vi "Hi_Port_TEST_SET.vi"(4 "itemiput":string, 5 "input":string, 6 "SEQ":i32, 7 "tpdata in":string[](array[string])) -> (3 "tpdata out":string[](array[string]))   [LabVIEW 2018]
panel:
  in  "Bar":bool
  out "布尔":bool
  in  "退出":bool
  out "out":string
  in  "Tab Control":enum32{"DataSetign", "RelaySeting"}(tab)
  in  "Address":string(combo)="PCI-1713"
  in  "Start board number":string(combo)="1"
  in  "Test Type":string(combo)="0"
  in  "Output Current Max.Spec":string="*" caption="MAX"
  in  "Output Current Min.Spec":string="*" caption="MIN"
  in  "延时时间(ms)2":string="0" caption="Delay Time (ms)"
  in  "备注":string
  in  "H 2":bool[](array[boolean])
  in  "L 2":bool[](array[boolean])
  in  "H":bool[](array[boolean])
  in  "L":bool[](array[boolean])
  in  "L 3":bool[](array[boolean])
  in  "H 3":bool[](array[boolean])
  in  "L 4":bool[](array[boolean])
  in  "H 4":bool[](array[boolean])
  in  "Cancel":bool
  in  "OK":bool
  # "EditTestData"
  # "9-16位输出"
  # "17-24位输出"
  # "25-32位输出"
  # "33-40位输出"
  # "41-48位输出"
  # "49-56位输出"
  # "57-64位输出"
  # "1-8位输出"
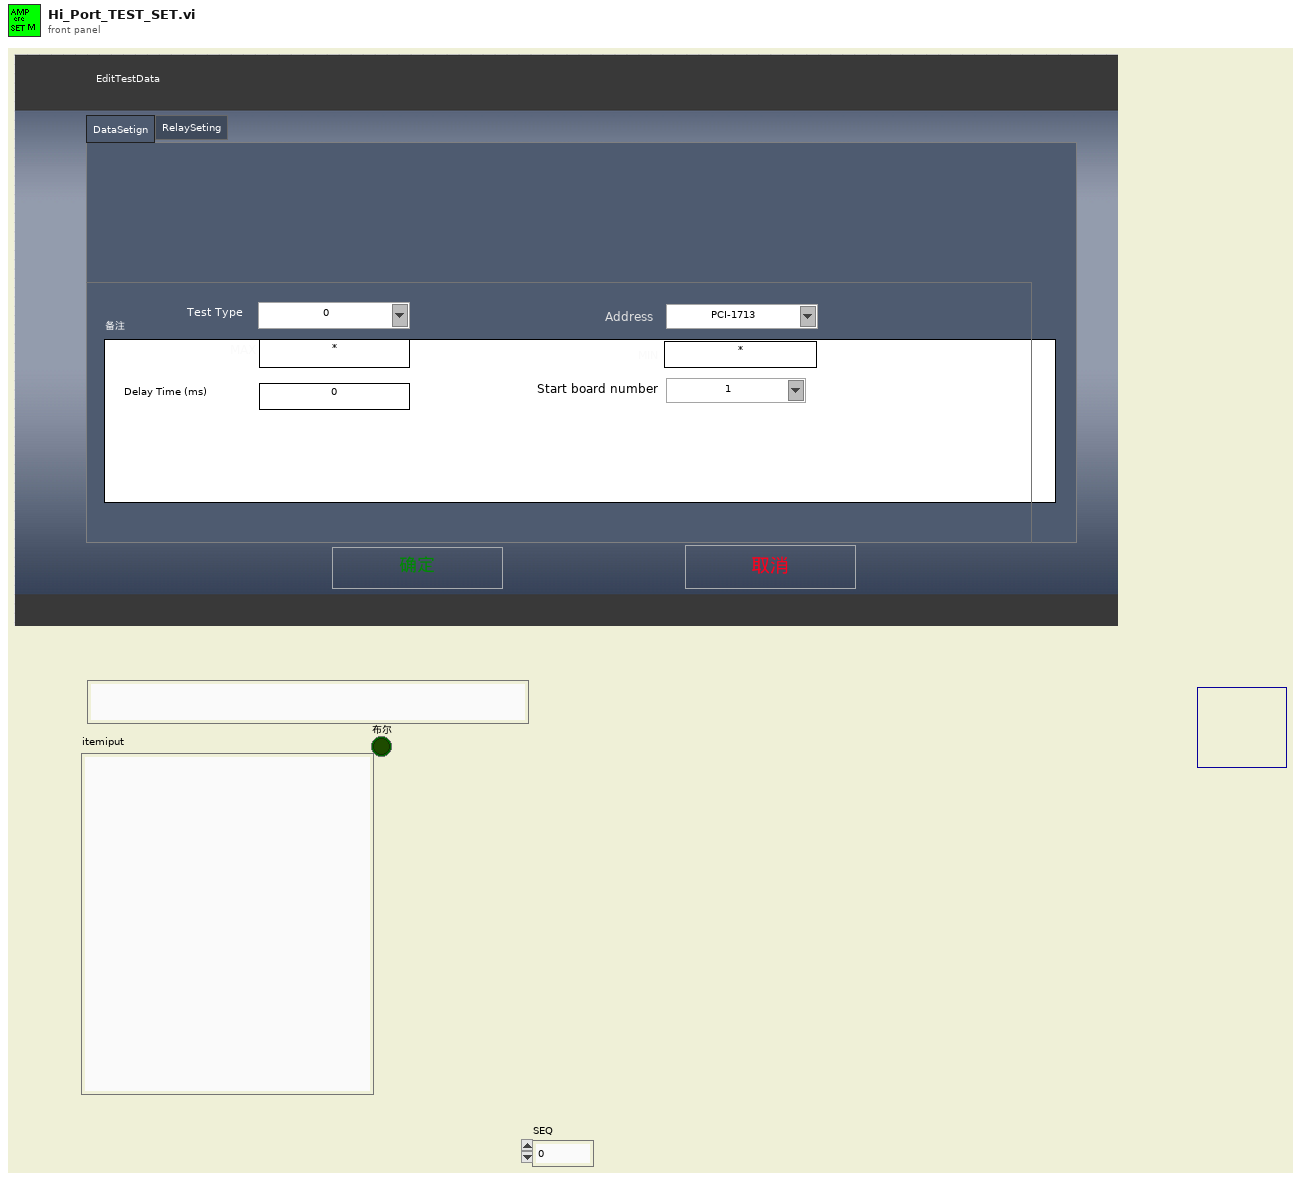
[diagram p1: front panel]
types:
  T1 = typedef "Window Refnum.ctl" = refnum<k1>
  T2 = typedef "Window Rectangle.ctl" = cluster{"left":i16, "top":i16, "right":i16, "bottom":i16}
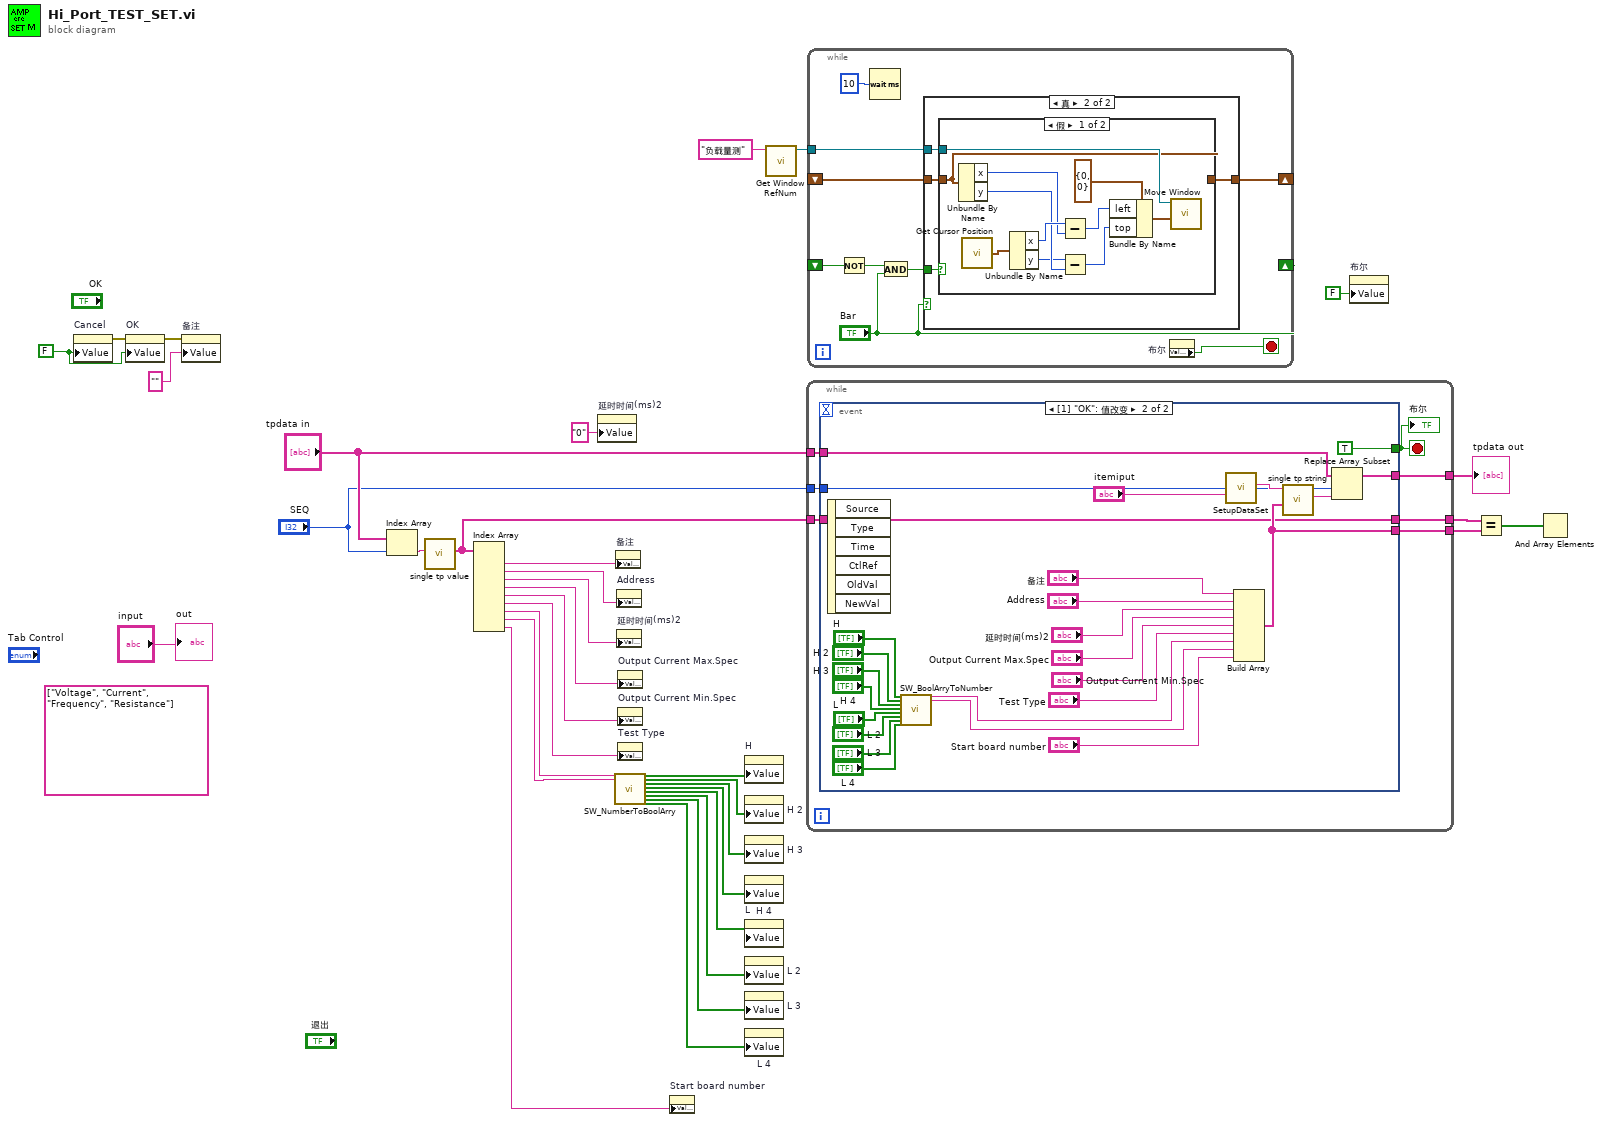
[diagram p0: block diagram]
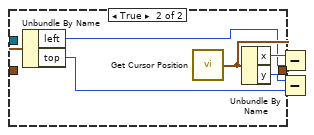
[diagram p3: hidden frame]
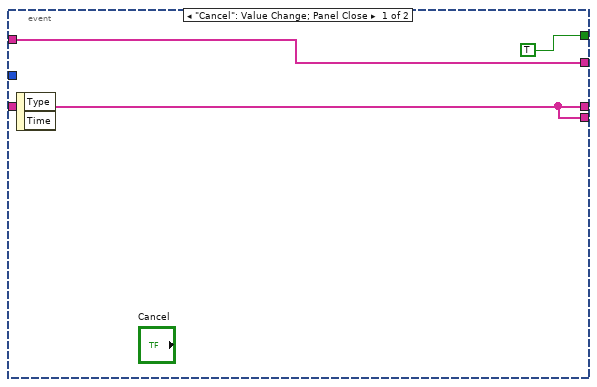
[diagram p4: hidden frame]
diagram:
  (unwired) string[] ["Voltage", "Current", "Frequency", "Resistance"]
  w31 = FALSE
  n1 = property on="Cancel" class="Bool (严格)"("Value"=w31) -> (error out=w33:errorcluster)  [unwired: 2 in, 1 out]
  n2 = property on="OK" class="Bool (严格)"(error in=w33, "Value"=w31) -> (error out=w32:errorcluster)  [unwired: 1 in, 1 out]
  n3 = property on="备注" class="Str"(error in=w32, "Value"="") -> ()  [unwired: 1 in, 2 out]
  n4 = Index Array(array="tpdata in", index="SEQ") -> (element=w21:string)
  n5 = call "single tp value.vi"("single tp data"=w21) -> ("value"=w19:string[])  [unwired: 10 out]
  n6 = Index Array(array=w19) -> (element #1=w20:string, element #2=w22:string, element #3=w23:string, element #4=w24:string, element #5=w25:string, element #6=w26:string, element #7=w11:string, element #8=w10:string, element #9=w15:string)  [unwired: 9 in]
  n7 = property on="延时时间(ms)2" class="Str"("Value"="0" ("延时时间(ms)2")) -> ()  [unwired: 2 in, 2 out]
  n8 = call "SW_NumberToBoolArry.vi"("L STR"=w11, "H STR"=w10) -> ("H1"=w9:bool[], "H2"=w8:bool[], "H3"=w7:bool[], "H4"=w6:bool[], "L1"=w5:bool[], "L2"=w4:bool[], "L3"=w3:bool[], "L4"=w2:bool[])  [unwired: 18 in]
  n9 = property on="备注" class="Str"("Value"=w20) -> ()  [unwired: 2 in, 2 out]
  n10 = property on="Address" class="CmbBox"("Value"=w22) -> ()  [unwired: 2 in, 2 out]
  n11 = property on="延时时间(ms)2" class="Str"("Value"=w23) -> ()  [unwired: 2 in, 2 out]
  n12 = property on="Output Current Max.Spec" class="Str"("Value"=w24) -> ()  [unwired: 2 in, 2 out]
  n13 = property on="Output Current Min.Spec" class="Str"("Value"=w25) -> ()  [unwired: 2 in, 2 out]
  n14 = property on="Test Type" class="CmbBox"("Value"=w26) -> ()  [unwired: 2 in, 2 out]
  n15 = property on="Start board number" class="CmbBox"("Value"=w15) -> ()  [unwired: 2 in, 2 out]
  n16 = property on="H" class="Arr (严格)"("Value"=w9) -> ()  [unwired: 2 in, 2 out]
  n17 = property on="H 2" class="Arr (严格)"("Value"=w8) -> ()  [unwired: 2 in, 2 out]
  n18 = property on="H 3" class="Arr (严格)"("Value"=w7) -> ()  [unwired: 2 in, 2 out]
  n19 = property on="H 4" class="Arr (严格)"("Value"=w6) -> ()  [unwired: 2 in, 2 out]
  n20 = property on="L" class="Arr (严格)"("Value"=w5) -> ()  [unwired: 2 in, 2 out]
  n21 = property on="L 2" class="Arr (严格)"("Value"=w4) -> ()  [unwired: 2 in, 2 out]
  n22 = property on="L 3" class="Arr (严格)"("Value"=w3) -> ()  [unwired: 2 in, 2 out]
  n23 = property on="L 4" class="Arr (严格)"("Value"=w2) -> ()  [unwired: 2 in, 2 out]
  n24 = call "Get Window RefNum.vi"("window name (\"\")"="负载量测" ("window name (\"\")")) -> ("window refnum (NaWR)"=w13:T1)  [unwired: 1 in, 7 out]
  n25 = while {
    tunnel: "tpdata in" -> [w40]
    tunnel: [w39] -> w28
    tunnel: "SEQ" -> [w38]
    tunnel: [w37] -> w27
    tunnel: w19 -> [w36]
    tunnel: [w35] -> w30
    stop <- w41 stop-if-true
    n26 = event shown="[1] \"OK\": 值改变" {
      selector: _ -> [_ _]
      dyn-events: _ -> [_ _]
      timeout: _ -> [_ _]
      tunnel: [TRUE TRUE] -> w41
      tunnel: [w43 w66] -> w39
      tunnel: w40 -> [w43 w67]
      tunnel: w38 -> [_ w65]
      tunnel: [w42 w63] -> w37
      tunnel: w36 -> [w42 w62]
      tunnel: [w42 w62] -> w35
      event "Cancel": Value Change; Panel Close {
        n27 = event-data() -> ()  [unwired: 3 out]
      }
      event "OK": Value Change {
        n28 = event-data() -> ()  [unwired: 7 out]
        n29 = call "SW_BoolArryToNumber.vi"("L1"="H", "L 2"="H 2", "L 3"="H 3", "L 4"="H 4", "L 5"="L", "L 6"="L 2", "L 7"="L 3", "L 8"="L 4") -> ("H"=w45:string, "L"=w46:string)  [unwired: 18 in]
        n30 = call "SetupDataSet.vi"("字符串"="itemiput") -> ("item data"=w69:string)  [unwired: 10 in]
        n31 = Build Array("备注", "Address", "延时时间(ms)2", "Output Current Max.Spec", "Output Current Min.Spec", "Test Type", w45, w46, "Start board number") -> (w63:string[])
        n32 = call "single tp string.vi"("value in"=w63, "oringnal defult tp data"=w69) -> ("new single tp data out"=w68:string)  [unwired: 9 out]
        n33 = Replace Array Subset(array=w67, new element=w68, index=w65) -> (w66:string[])
      }
    }
    "布尔" <- w41
  }
  "tpdata out" <- w28
  n34 = while {
    shift-left: _ -> [w73]
    shift-right: [w74] -> _
    shift-left: _ -> [w77]
    shift-right: ["Bar"] -> _
    tunnel: w13 -> [w78]
    stop <- w71 stop-if-true
    n35 = Not(x=w77) -> (.not. x?=w76:bool)
    n36 = Wait (ms)(milliseconds to wait=u32 10) -> ()  [unwired: 1 out]
    n37 = And(x=w76, y="Bar") -> (x .and. y?=w72:bool)
    n38 = case shown="真" "Bar" {
      tunnel: w78 -> [_ w84]
      tunnel: [w80 w83] -> w74
      tunnel: w73 -> [w80 w81]
      tunnel: w72 -> [_ w82]
      frame False {
      }
      frame True {
        n39 = case shown="假" w82 {
          tunnel: w84 -> [w90 w106]
          tunnel: [w85 w96] -> w83
          tunnel: w81 -> [w85 _]
          frame False {
            n40 = Unbundle By Name(w85) -> ("x"=w93:i16, "y"=w92:i16)
            n41 = call "Get Cursor Position.vi"() -> ("cursor position"=w95:cluster{"x":i16, "y":i16})
            n42 = Unbundle By Name(w95) -> ("x"=w94:i16, "y"=w91:i16)
            n43 = Subtract(x=w94, y=w93) -> (x-y=w87:i16)
            n44 = Subtract(x=w91, y=w92) -> (x-y=w88:i16)
            n45 = Bundle By Name(cluster=cluster{"left":i16, "top":i16} {"left"=0, "top"=0} ("new position (0,0)"), "left"=w87, "top"=w88) -> (w86:cluster{"left":i16, "top":i16})
            n46 = call "Move Window.vi"("new position (0,0)"=w86, "window refnum (NaWR)"=w90) -> ()  [unwired: 2 in, 4 out]
          }
          frame True {
            n47 = call "Get Window Rectangle.vi"("window refnum (NaWR)"=w106) -> ("window rect"=w105:T2)  [unwired: 1 in, 5 out]
            n48 = call "Extract Window Origin.vi"("window rect"=w105) -> ("window origin"=w104:cluster{"left":i16, "top":i16})  [unwired: 1 out]
            n49 = Unbundle By Name(w104) -> ("left"=w101:i16, "top"=w100:i16)
            n50 = call "Get Cursor Position.vi"() -> ("cursor position"=w103:cluster{"x":i16, "y":i16})
            n51 = Unbundle By Name(w103) -> ("x"=w102:i16, "y"=w99:i16)
            n52 = Subtract(x=w102, y=w101) -> (x-y=w97:i16)
            n53 = Subtract(x=w99, y=w100) -> (x-y=w98:i16)
            n54 = Bundle By Name(cluster=w103, "x"=w97, "y"=w98) -> (w96:cluster{"x":i16, "y":i16})
          }
        }
      }
    }
    n55 = property on="布尔" class="Bool (严格)"() -> ("Value"=w71:bool)  [unwired: 2 in, 2 out]
  }
  n56 = property on="布尔" class="Bool (严格)"("Value"=FALSE ("布尔")) -> ()  [unwired: 2 in, 2 out]
  n57 = Equal?(x=w30, y=w27) -> (x = y?=w29:bool[])
  n58 = And Array Elements(Boolean array=w29) -> ()  [unwired: 1 out]
  "out" <- "input"
